vi "Single VI Decode.vi"(11 "filename (use dialog)":path) -> ()   [LabVIEW 2016]
uses:
  clFile/clFile.lvclass
  clLabview/clLabview.lvclass
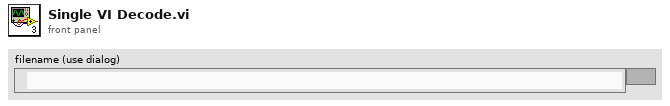
[diagram p1: front panel]
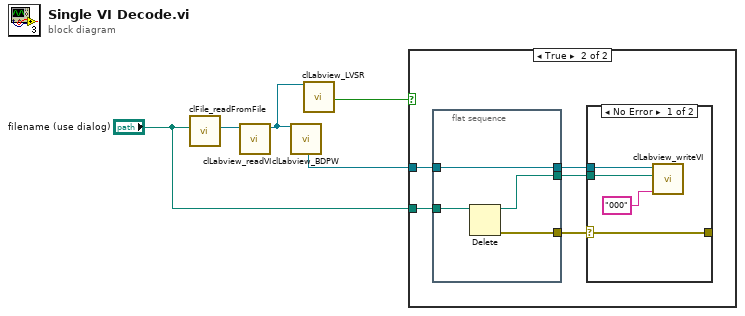
[diagram p0: block diagram]
diagram:
  n1 = call "clFile_readFromFile.vi"("file (use dialog)"="filename (use dialog)") -> ("clFileReader.lvclass"=w5:refnum<class "clFileReader.lvclass">)  [unwired: 1 in, 9 out]
  n2 = call "clLabview_readVI.vi"("vi_lib.lvlib:clFileReader.lvclass"=w5) -> ("vi_lib.lvlib:clLabview.lvclass 2"=w2:refnum<class "clLabview.lvclass">)  [unwired: 10 out]
  n3 = call "clLabview_BDPW.vi"("vi_lib.lvlib:clLabview.lvclass"=w2) -> ("vi_lib.lvlib:clLabview.lvclass [Out]"=w3:refnum<class "clLabview.lvclass">)  [unwired: 18 out]
  n4 = call "clLabview_LVSR.vi"("vi_lib.lvlib:clLabview.lvclass"=w2) -> ("File is protected?"=w1:bool)  [unwired: 18 out]
  n5 = case shown="True" w1 {
    tunnel: "filename (use dialog)" -> [_ w10]
    tunnel: w3 -> [_ w6]
    frame False {
    }
    frame True {
      n6 = flat-sequence {
        tunnel: w10 -> [w14]
        tunnel: [w13] -> w9
        tunnel: [w12] -> w8
        tunnel: [w11] -> w7
        tunnel: w6 -> [w11]
        frame #0 {
          n7 = Delete(path (use dialog)=w14) -> (deleted path=w13:path, error out=w12:errorcluster)  [unwired: 4 in, 1 out]
        }
      }
      n8 = case shown="No Error" w8 {
        selector: w8 -> [w15 w19]
        tunnel: w7 -> [w18 _]
        tunnel: w9 -> [w16 _]
        tunnel: [w15 w19] -> _
        frame No Error {
          n9 = call "clLabview_writeVI.vi"("vi_lib.lvlib:clLabview.lvclass"=w18, "filename (use dialog)"=w16, "new Password"="000") -> ()  [unwired: 8 out]
        }
        frame Error {
        }
      }
    }
  }
